vi "SNRPowerGainStructure_ChangePowerFreq.vi"(8 "RFSA Analyze Input":T2={"Published Data Id"=[], "frequency range"={"start frequency"=-1.0, "stop frequency"=-1.0}, "Power Level"=0.0}, 9 "RFSG Input":T3={"LO configure setting"={"Carrier Frequency (Hz)"=5180000000.0, "Power Level(dBm)"=-10.0, "External Attenuation (dB)"=0.0}, "Port"=""} {"LO configure setting"."Carrier Frequency (Hz)" format="%#_6p"}, 10 "RFSA Input":T1 {"reference level (dBm)" format="%.2f"}, 11 "Semiconductor Module Context":T4) -> (0 "error out":errorcluster)   [LabVIEW 2014]
uses:
  <vilib>/NI_TestStand_SemiconductorModule/NI_TestStand_Semiconductor_Module.lvlibp/PinMap/General/SemiconductorModuleContext.ctl
  Control/RFSG Input.ctl
  Control/RFSA Analyze Input.ctl
  Control/RFSA Input.ctl
  Control/Quene Type_RFSA.ctl
  <vilib>/NI_TestStand_SemiconductorModule/NI_TestStand_Semiconductor_Module.lvlibp/PinMap/PinQueryContext/MultiplePinMultipleSessionQueryContext/MultiplePinMultipleSessionQueryContext.lvclass
  <vilib>/NI_TestStand_SemiconductorModule/NI_TestStand_Semiconductor_Module.lvlibp/PinMap/RF/RFPM/PinToNIRFPMSessions.vi
  <vilib>/NI_TestStand_SemiconductorModule/NI_TestStand_Semiconductor_Module.lvlibp
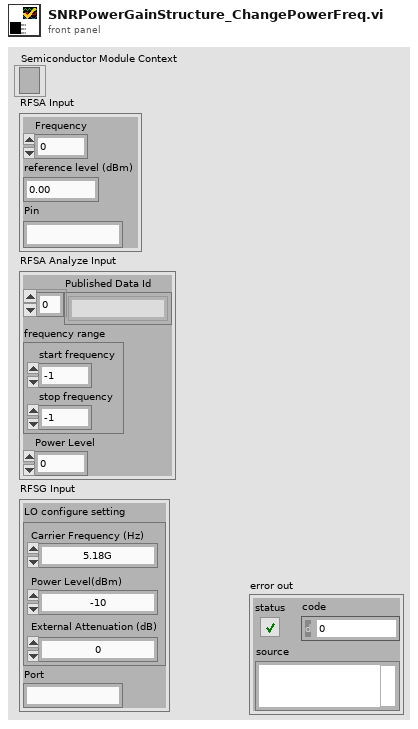
[diagram p1: front panel]
types:
  T1 = typedef "RFSA Input.ctl" = cluster{"Frequency":dbl, "reference level (dBm)":dbl, "Pin":string}
  T2 = typedef "RFSA Analyze Input.ctl" = cluster{"Published Data Id":string[], "frequency range":cluster{"start frequency":dbl, "stop frequency":dbl}, "Power Level":dbl}
  T3 = typedef "RFSG Input.ctl" = cluster{"LO configure setting":cluster{"Carrier Frequency (Hz)":dbl, "Power Level(dBm)":dbl, "External Attenuation (dB)":dbl}, "Port":string}
  T4 = typedef "NI_TestStand_Semiconductor_Module.lvlibp/SemiconductorModuleContext.ctl" = refnum<k7>
  T5 = typedef "Quene Type_RFSA.ctl" = cluster{"Actiion":enum16{"Exit", "Analyze"}, "Pin Query Context":refnum<class "MultiplePinMultipleSessionQueryContext.lvclass">, "Semiconductor Module Context":T4, "power spectrum":cluster{"f0":dbl, "df":dbl, "data":dbl[]}, "error constant":errorcluster}
  T6 = cluster{"Carrier Frequency (Hz)":dbl, "Power Level(dBm)":dbl, "External Attenuation (dB)":dbl}
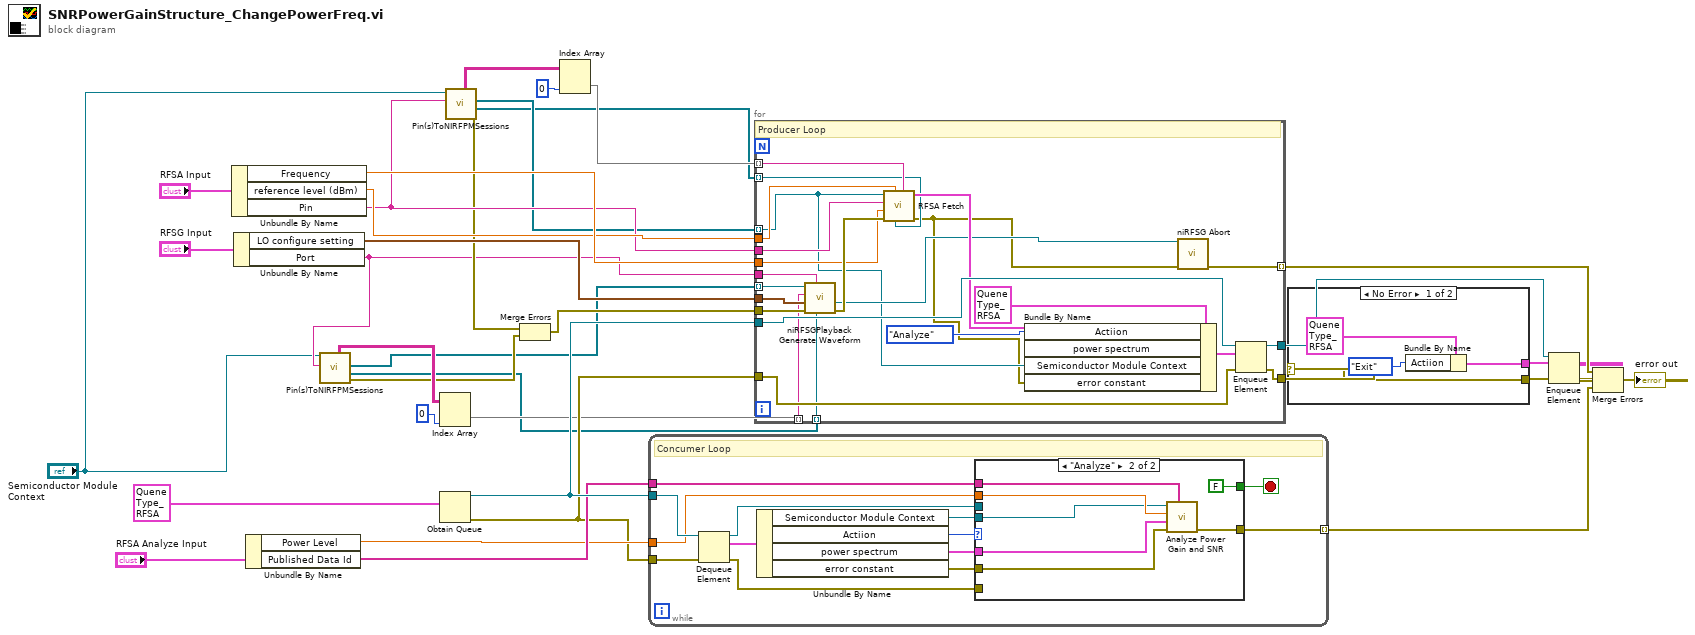
[diagram p0: block diagram]
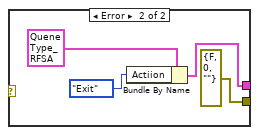
[diagram p2: hidden frame]
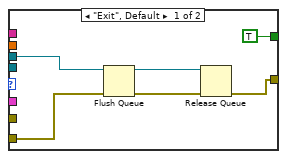
[diagram p3: hidden frame]
diagram:
  n1 = Unbundle By Name("RFSA Input") -> ("Frequency"=w18:dbl, "reference level (dBm)"=w17:dbl, "Pin"=w14:string)
  n2 = Unbundle By Name("RFSG Input") -> ("LO configure setting"=w33:T6, "Port"=w8:string)
  n3 = Unbundle By Name("RFSA Analyze Input") -> ("Power Level"=w28:dbl, "Published Data Id"=w29:string[])
  n4 = call-poly <vilib>:"Pin(s)ToNIRFPMSessions.vi"("Pin"=w8, "Semiconductor Module Context"="Semiconductor Module Context") -> ("error out"=w6:errorcluster, "Instrument Sessions"=w3:refnum<k15>[], "Semiconductor Module Contexts"=w5:refnum<k7>[], "Ports List"=w9:string[][])  [unwired: 4 in, 2 out]
  n5 = Index Array(array=w9, index (col)=0) -> (element=w4:string[])  [unwired: 1 in]
  n6 = Obtain Queue(element data type=T5 {"Actiion"=enum."Analyze", "Pin Query Context"=refnum, "Semiconductor Module Context"=refnum, "power spectrum"={"f0"=0.0, "df"=0.0, "data"=[]}, "error constant"={"status"=FALSE, "code"=0, "source"=""}}) -> (queue out=w31:refnum<queue>, error out=w23:errorcluster)  [unwired: 4 in, 1 out]
  n7 = call-poly <vilib>:"Pin(s)ToNIRFPMSessions.vi"("Pin"=w14, "Semiconductor Module Context"="Semiconductor Module Context") -> ("error out"=w12:errorcluster, "Instrument Sessions"=w1:refnum<k15>[], "Semiconductor Module Contexts"=w13:refnum<k7>[], "Ports List"=w16:string[][])  [unwired: 4 in, 2 out]
  n8 = Merge Errors(w12, w6) -> (w11:errorcluster)
  n9 = Index Array(array=w16, index (col)=0 ("index (row)")) -> (element=w2:string[])  [unwired: 1 in]
  n10 = while {
    tunnel: w31 -> [w48]
    tunnel: w29 -> [w42]
    tunnel: w28 -> [w41]
    tunnel: w23 -> [w47]
    tunnel: [w38] -> w25 mode=indexing
    stop <- w44 stop-if-true
    # "Concumer Loop"
    n11 = Dequeue Element(queue=w48, error in (no error)=w47) -> (queue out=w40:refnum<queue>, element=w46:T5, error out=w39:errorcluster)  [unwired: 1 in, 1 out]
    n12 = Unbundle By Name(w46) -> ("Semiconductor Module Context"=w37:T4, "Actiion"=w45:enum16{"Exit", "Analyze"}, "power spectrum"=w43:cluster{"f0":dbl, "df":dbl, "data":dbl[]}, "error constant"=w36:errorcluster)
    n13 = case shown="\"Analyze\"" w45 {
      tunnel: [TRUE FALSE] -> w44
      tunnel: w43 -> [_ w60]
      tunnel: w42 -> [_ w59]
      tunnel: w41 -> [_ w57]
      tunnel: w40 -> [w51 _]
      tunnel: w39 -> [w50 _]
      tunnel: [w49 w58] -> w38
      tunnel: w37 -> [_ w56]
      tunnel: w36 -> [_ w55]
      frame "Exit", Default {
        n14 = Flush Queue(queue=w51, error in (no error)=w50) -> (queue out=w53:refnum<queue>, error out=w52:errorcluster)  [unwired: 1 out]
        n15 = Release Queue(queue=w53, error in (no error)=w52) -> (error out=w49:errorcluster)  [unwired: 1 in, 2 out]
      }
      frame "Analyze" {
        n16 = call "Analyze Power Gain and SNR.vi"("Published Data Id"=w59, "error in (no error)"=w55, "power spectrum"=w60, "power level (dBm)"=w57, "Automation Refnum in"=w56) -> ("error out"=w58:errorcluster)  [unwired: 4 in, 2 out]
      }
    }
  }
  n17 = for {
    tunnel: w5 -> [w84] mode=indexing
    tunnel: w33 -> [w83]
    tunnel: w8 -> [w82]
    tunnel: w31 -> [w80]
    tunnel: [w74] -> w32
    tunnel: w11 -> [w85]
    tunnel: [w65] -> w24 mode=indexing
    tunnel: w23 -> [w73]
    tunnel: [w75] -> w22
    tunnel: w18 -> [w72]
    tunnel: w17 -> [w71]
    tunnel: w14 -> [w70]
    tunnel: w13 -> [w63] mode=indexing
    tunnel: w4 -> [w69] mode=indexing
    tunnel: w3 -> [w68] mode=indexing
    tunnel: w2 -> [w67] mode=indexing
    tunnel: w1 -> [w66] mode=indexing
    # "Producer Loop"
    n18 = call "niRFSGPlayback Generate Waveform.vi"("instrument handle"=w68, "Port"=w82, "error in (no error)"=w85, "LO configure setting"=w83, "TX port"=w69, "TSM Context"=w84) -> ("error out"=w81:errorcluster, "instrument handle out"=w64:refnum<k15>)  [unwired: 4 in]
    n19 = call "RFSA Fetch.vi"("RX Port"=w67, "instrument handle"=w66, "reference level (dBm)"=w71, "error in (no error)"=w81, "Frequency"=w72, "Pin"=w70, "Semiconductor Module Context"=w63) -> ("error out"=w62:errorcluster, "power spectrum"=w78:cluster{"f0":dbl, "df":dbl, "data":dbl[]})  [unwired: 3 in]
    n20 = Bundle By Name(cluster=T5 {"Actiion"=enum."Exit", "Pin Query Context"=refnum, "Semiconductor Module Context"=refnum, "power spectrum"={"f0"=0.0, "df"=0.0, "data"=[]}, "error constant"={"status"=FALSE, "code"=0, "source"=""}}, "Actiion"=enum16{"Exit", "Analyze"}."Analyze", "power spectrum"=w78, "Semiconductor Module Context"=w63, "error constant"=w62) -> (w76:T5)
    n21 = call <instrlib>:"niRFSG Abort.vi"("instrument handle"=w64, "error in"=w62) -> ("error out"=w65:errorcluster)  [unwired: 12 in, 1 out]
    n22 = Enqueue Element(queue=w80, element=w76, error in (no error)=w73) -> (queue out=w74:refnum<queue>, error out=w75:errorcluster)  [unwired: 1 in, 1 out]
  }
  n23 = case shown="No Error" w22 {
    selector: w22 -> [w86 _]
    tunnel: [w87 w90] -> w21
    tunnel: [w86 errorcluster {"status"=FALSE, "code"=0, "source"=""} ("error IO")] -> w20
    frame No Error {
      n24 = Bundle By Name(cluster=T5 {"Actiion"=enum."Analyze", "Pin Query Context"=refnum, "Semiconductor Module Context"=refnum, "power spectrum"={"f0"=0.0, "df"=0.0, "data"=[]}, "error constant"={"status"=FALSE, "code"=0, "source"=""}}, "Actiion"=enum16{"Exit", "Analyze"}."Exit") -> (w87:T5)
    }
    frame Error {
      n25 = Bundle By Name(cluster=T5 {"Actiion"=enum."Analyze", "Pin Query Context"=refnum, "Semiconductor Module Context"=refnum, "power spectrum"={"f0"=0.0, "df"=0.0, "data"=[]}, "error constant"={"status"=FALSE, "code"=0, "source"=""}}, "Actiion"=enum16{"Exit", "Analyze"}."Exit") -> (w90:T5)
    }
  }
  n26 = Enqueue Element(queue=w32, element=w21, error in (no error)=w20) -> (error out=w26:errorcluster)  [unwired: 1 in, 2 out]
  n27 = Merge Errors(w24, w26, w25) -> (→"error out":errorcluster)
